vi "Write New Send Method.vi"(10 "New Send Method":path, 11 "Concrete Send Builder in":refnum<class "Concrete Send Builder.lvclass">) -> (3 "Concrete Send Builder out":refnum<class "Concrete Send Builder.lvclass">)   [LabVIEW 2020, in "Message Maker.lvlib" / "Concrete Send Builder.lvclass"]
uses:
  Concrete Send Builder.lvclass
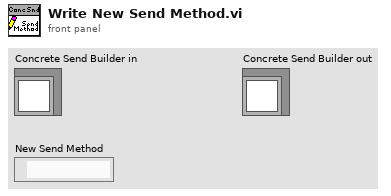
[diagram p1: front panel]
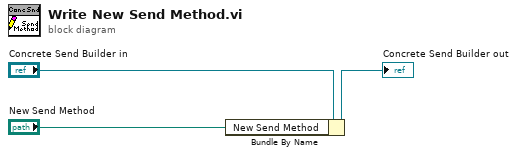
[diagram p0: block diagram]
diagram:
  n1 = Bundle By Name(cluster="Concrete Send Builder in", "New Send Method"="New Send Method") -> (→"Concrete Send Builder out":refnum<class "Concrete Send Builder.lvclass">)
